vi "Clear All Items.vi"(8 "错误输入":errorcluster, 11 "Listbox Ref":refnum<vi>) -> (0 "错误输出":errorcluster, 3 "Dup Listbox Ref":refnum<vi>)   [LabVIEW 2012, in "Listbox Tool.lvlib"]
uses:
  Listbox Tool.lvlib
  Custom Type/Read and Write Mode.ctl
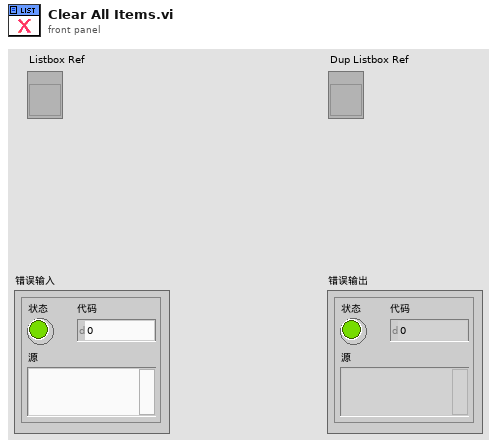
[diagram p1: front panel]
types:
  T1 = typedef "Listbox Tool.lvlib/Read and Write Mode.ctl" = enum16{"Read", "Write"}
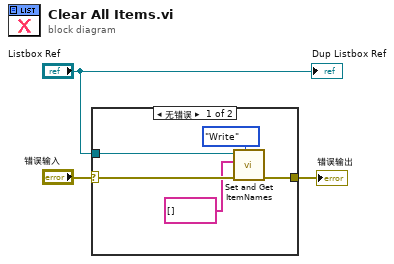
[diagram p0: block diagram]
diagram:
  n1 = case shown="无错误" "错误输入" {
    selector: "错误输入" -> [w5 w9]
    tunnel: "Listbox Ref" -> [w6 _]
    tunnel: [w7 w9] -> w1
    frame No Error {
      n2 = call "Set and Get ItemNames.vi"("Mode"=Read_and_Write_Mode."Write", "错误输入"=w5, "ItemNames In"=string[] [], "Listbox Ref"=w6) -> ("错误输出"=w7:errorcluster)  [unwired: 5 in, 2 out]
    }
    frame Error {
    }
  }
  "错误输出" <- w1
  "Dup Listbox Ref" <- "Listbox Ref"
